vi "Roots Classification.vi"(9 "tolerance for conjugate pair":dbl=1e-07, 10 "tolerance for real roots":dbl=1e-10, 11 "Roots":cdb[](array[numeric])) -> (0 "error":i32, 1 "Pure Complex Roots":cdb[](array[numeric]), 2 "Complex Pair Roots":cdb[](array[numeric]), 3 "Real Roots":dbl[](array[numeric]))   [LabVIEW 2024, in "NI_AALPro.lvlib"]
doc: "<p>Classifies <strong>Roots</strong> into real, complex conjugate pair, and pure complex roots.</p>"
uses:
  NI_AALPro.lvlib
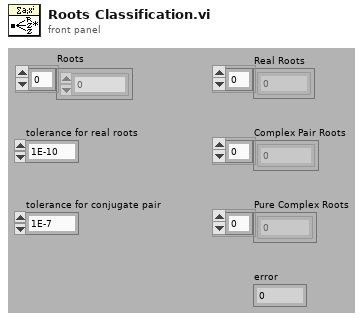
[diagram p1: front panel]
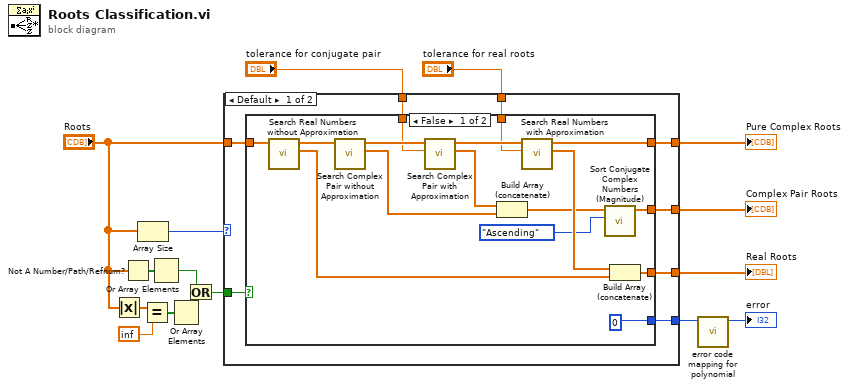
[diagram p0: block diagram]
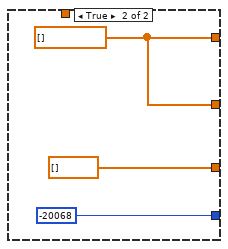
[diagram p2: hidden frame]
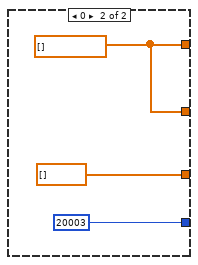
[diagram p3: hidden frame]
diagram:
  n1 = Absolute Value(x="Roots") -> (abs(x)=w8:dbl[])
  n2 = Not A Number/Path/Refnum?(number/path/refnum="Roots") -> (NaN/Path/Refnum?=w10:bool[])
  n3 = Array Size(array="Roots") -> (size(s)=w11:i32)
  n4 = Equal?(x=w8, y=inf) -> (x = y?=w5:bool[])
  n5 = Or Array Elements(Boolean array=w10) -> (logical OR=w4:bool)
  n6 = Or Array Elements(Boolean array=w5) -> (logical OR=w3:bool)
  n7 = Or(x=w4, y=w3) -> (x .or. y?=w6:bool)
  n8 = case shown="Default" w11 {
    tunnel: [w18 w45] -> w16
    tunnel: "Roots" -> [w24 _]
    tunnel: [w23 w45] -> w15
    tunnel: [w22 dbl[] [] ("BDL")] -> w14
    tunnel: "tolerance for conjugate pair" -> [w21 _]
    tunnel: "tolerance for real roots" -> [w20 _]
    tunnel: [w19 20003 ("empty array")] -> w2
    tunnel: w6 -> [w17 _]
    frame Default {
      n9 = case shown="False" w17 {
        tunnel: w24 -> [w37 _]
        tunnel: [w34 w43] -> w23
        tunnel: [w31 dbl[] []] -> w22
        tunnel: w21 -> [w30 _]
        tunnel: w20 -> [w29 _]
        tunnel: [0 -20068 ("MatrixInfNanErr")] -> w19
        tunnel: [w26 w43] -> w18
        frame False {
          n10 = call "Search Real Numbers without Approximation.vi"("Complex Numbers In"=w37) -> ("Real Numbers"=w32:dbl[], "Complex Numbers Out"=w36:cdb[])  [unwired: 9 in]
          n11 = call "Search Complex Pair without Approximation.vi"("Complex Numbers"=w36) -> ("Complex Pair Numbers"=w39:cdb[], "Pure Complex Numbers"=w40:cdb[])  [unwired: 9 in]
          n12 = call "Search Complex Pair with Approximation.vi"("tolerance for complex pair"=w30, "Complex Numbers"=w40) -> ("Complex Pair Numbers"=w38:cdb[], "Pure Complex Numbers"=w35:cdb[])  [unwired: 8 in]
          n13 = Build Array (concatenate)(w38, w39) -> (w27:cdb[])
          n14 = call "Search Real Numbers with Approximation.vi"("tolerance for real numbers"=w29, "Numbers"=w35) -> ("Real Numbers"=w33:dbl[], "Complex Numbers"=w34:cdb[])  [unwired: 8 in]
          n15 = call "Sort Conjugate Complex Numbers (Magnitude).vi"("Order"=enum16{"Ascending", "Descending"}."Ascending", "Conjugate Complex Numbers"=w27) -> ("Sorted Conjugate Complex Numbers"=w26:cdb[])  [unwired: 9 in]
          n16 = Build Array (concatenate)(w33, w32) -> (w31:dbl[])
        }
        frame True {
          w43 = cdb[] [] ("Complex Numbers")
        }
      }
    }
    frame 0 {
      w45 = cdb[] [] ("CDB")
    }
  }
  "Pure Complex Roots" <- w15
  "Complex Pair Roots" <- w16
  "Real Roots" <- w14
  n17 = call "error code mapping for polynomial.vi"("error in"=w2) -> ("error out"=→"error":i32)  [unwired: 10 in]
